vi "Dac_Voice_coil_Camera_trigger.vi"(0 "Voice coil function generation":T1={"File to read"=path "C:/Users/lpk27/Documents/pan-ASLMsynched/pan-ASLM/Calibration files/newcalibration_voice coil input_25msflyback.txt", "Image acquisition time (ms)"=1000.0, "Flyback time (ms)"=25.0}, 5 "error in":errorcluster, 9 "DAQ setup":enum16{"Test setup", "Microscope"}(ring)) -> ()   [LabVIEW 2020]
uses:
  typedefs/typedef_voice_coil_function_generation.ctl
  <vilib>/DAQmx/write.llb/DAQmx Write (Analog Wfm 1Chan NSamp).vi
  <vilib>/Utility/file.llb/Read Delimited Spreadsheet (DBL).vi
  <vilib>/DAQmx/create/channels.llb/DAQmx Create Channel (AO-Voltage-Basic).vi
  <vilib>/DAQmx/configure/timing.llb/DAQmx Timing (Sample Clock).vi
  <vilib>/DAQmx/miscellaneous.llb/DAQmx Fill In Error Info.vi
  <vilib>/DAQmx/create/channels.llb/DAQmx Create Channel (CO-Pulse Generation-Ticks).vi
  <vilib>/DAQmx/configure/timing.llb/DAQmx Timing (Implicit).vi
  <vilib>/DAQmx/create/channels.llb/DAQmx Create Channel (CO-Pulse Generation-Frequency).vi
  Global stop DAQ.vi
  <resource>/objmgr/daqmx.rc
panel:
  out "error out 4":errorcluster
  out "error out 3":errorcluster
  out "LabVIEW generated Sawtooth input (blue) and Camera trigger (red)":waveform(dbl)(graph)={"t0"=timestamp(0 s since 1904-01-01), "dt"=1.0, "Y"=array[3075 elements]}
  out "# Samples written per channel":u32=3075
  out "actual frequency":dbl=1000.0
  in  "stop":bool
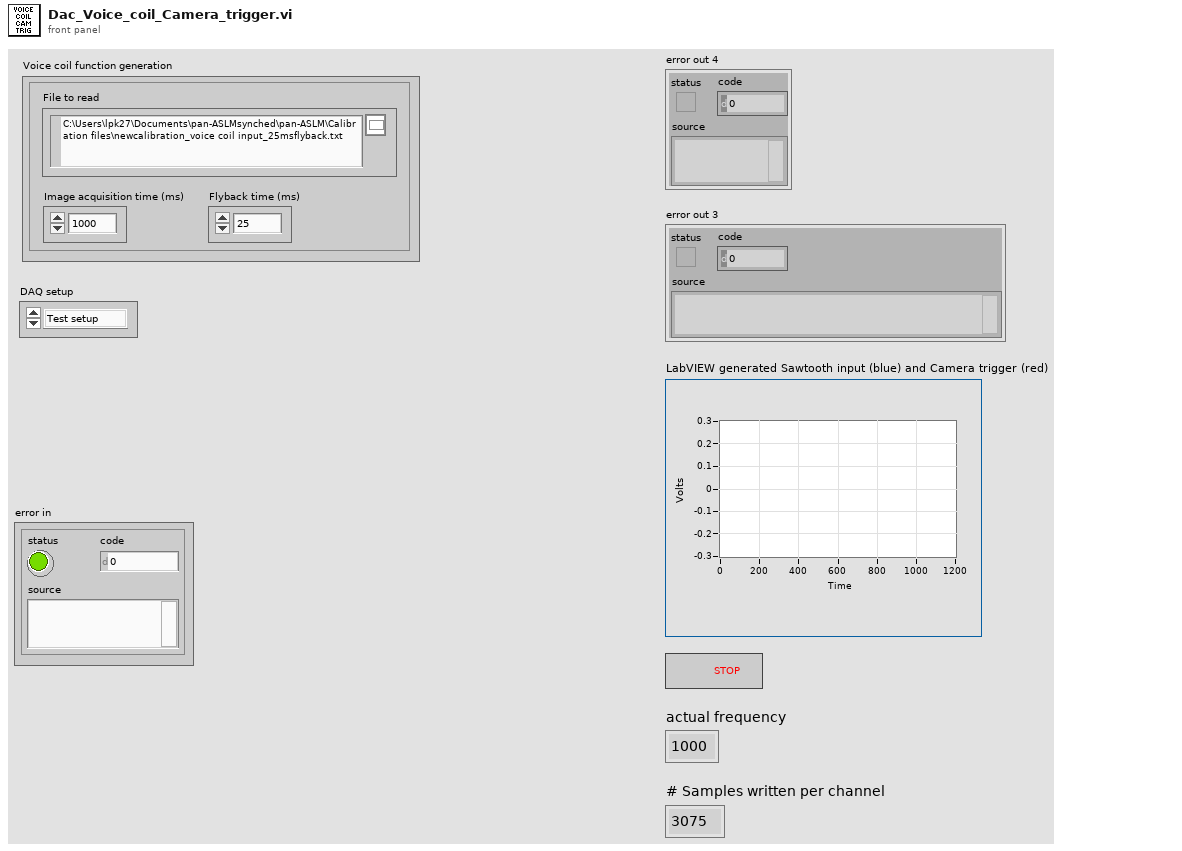
[diagram p1: front panel]
types:
  T1 = typedef "typedef_voice_coil_function_generation.ctl" = cluster{"File to read":path, "Image acquisition time (ms)":dbl, "Flyback time (ms)":dbl}
  T2 = typedef "DAQ_channel_typedef.ctl" = cluster{"CO.Pulse.Term":tag, "Voice coil analog output":tag, "counter":tag, "CO.Pulse.Term 2":tag, "AOTF lines":tag, "counter 2":tag, "CO.Pulse.Term 3":tag, "counter 3":tag}
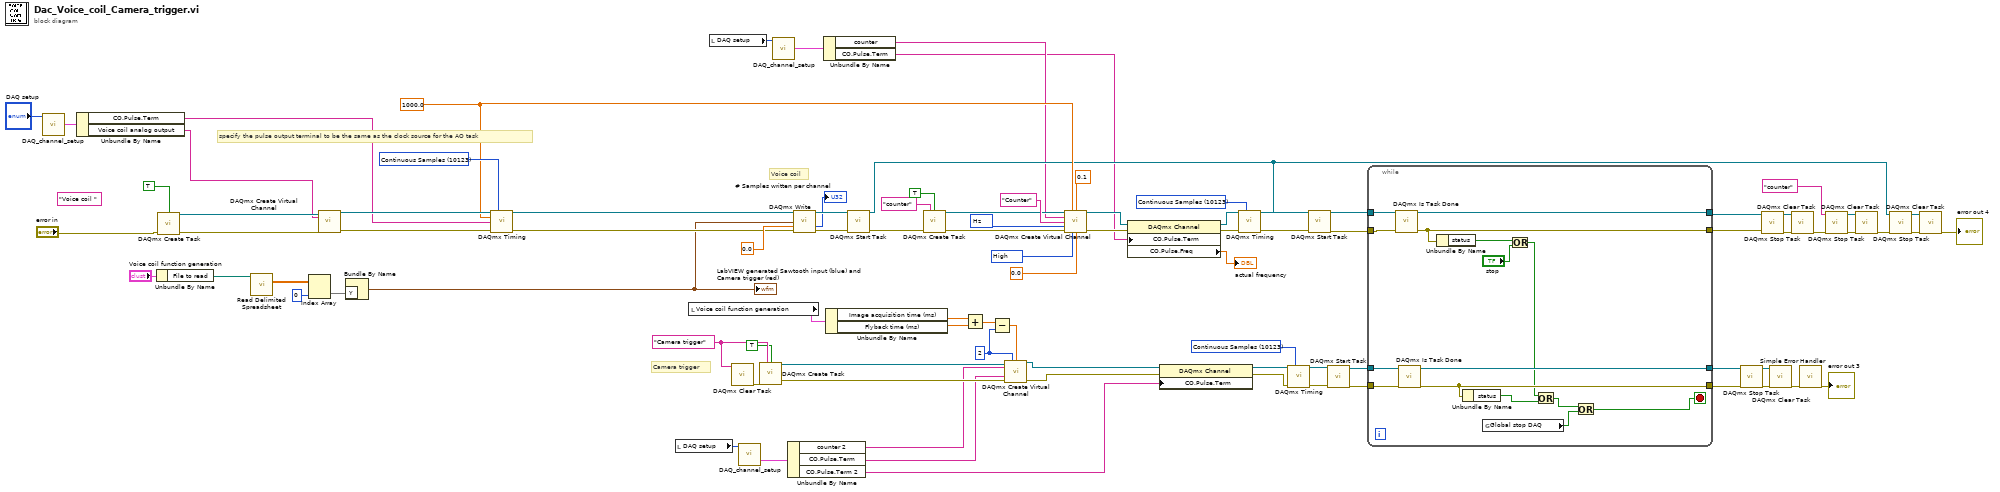
[diagram p0: block diagram]
diagram:
  w20 = "Camera trigger" ("new task name")
  (unwired) "Voice coil " ("new task name")
  w51 = u32 2 ("high ticks")
  w61 = 10123 items=["Finite Samples"=10178, "Continuous Samples"=10123, "Hardware Timed Single Point"=12522] ("sample mode")
  w73 = 10192 items=["High"=10192, "Low"=10214] ("idle state")
  w74 = 10373 items=["Hz"=10373] ("units")
  w67 = 10123 items=["Finite Samples"=10178, "Continuous Samples"=10123, "Hardware Timed Single Point"=12522] ("sample mode")
  w66 = 1000.0 ("rate")
  w89 = 10123 items=["Finite Samples"=10178, "Continuous Samples"=10123, "Hardware Timed Single Point"=12522] ("sample mode")
  # "Camera trigger"
  # "Voice coil"
  # "specify the pulse output terminal to be the same as the clock source for the AO task"
  n1 = call "DAQ_channel_setup.vi"("Text Ring"="DAQ setup") -> ("DAQ channels OUT"=w14:T2)  [unwired: 10 in]
  n2 = Unbundle By Name(w14) -> ("CO.Pulse.Term"=w4:tag, "Voice coil analog output"=w13:tag)
  n3 = Unbundle By Name("Voice coil function generation") -> ("File to read"=w44:path)
  n4 = call <vilib>:"DAQmx Create Task.vi"("auto cleanup"=TRUE, "error in"="error in") -> ("task out"=w49:refnum<k21>, "error out"=w48:errorcluster)  [unwired: 12 in]
  n5 = call-poly <vilib>:"Read Delimited Spreadsheet.vi"("file path (dialog if empty)"=w44) -> ("all rows"=w58:dbl[][])  [unwired: 9 in, 5 out]
  n6 = Index Array(array=w58, index (col)=0 ("disabled index (col)")) -> (element=w56:dbl[])  [unwired: 1 in]
  n7 = call-poly <vilib>:"DAQmx Create Virtual Channel.vi"("task in"=w49, "physical channels"=w13, "error in"=w48) -> ("task out"=w91:refnum<k21>, "error out"=w90:errorcluster)  [unwired: 11 in]
  n8 = Bundle By Name("Y"=w56) -> (w55:waveform(dbl))  [unwired: 1 in]
  "LabVIEW generated Sawtooth input (blue) and Camera trigger (red)" <- w55
  n9 = call-poly <vilib>:"DAQmx Timing.vi"("task/channels in"=w91, "sample mode"=w89, "rate"=w66, "source"=w4, "error in"=w90) -> ("task out"=w69:refnum<k21>, "error out"=w68:errorcluster)  [unwired: 9 in]
  n10 = local read "DAQ setup"() -> (w11:enum16{"Test setup", "Microscope"})
  n11 = local read "Voice coil function generation"() -> (w43:T1)
  n12 = local read "DAQ setup"() -> (w7:enum16{"Test setup", "Microscope"})
  n13 = call <vilib>:"DAQmx Clear Task.vi"("task in"=w20) -> ("error out"=w21:errorcluster)  [unwired: 14 in]
  n14 = call "DAQ_channel_setup.vi"("Text Ring"=w11) -> ("DAQ channels OUT"=w12:T2)  [unwired: 10 in]
  n15 = call <vilib>:"DAQmx Create Task.vi"("new task name"=w20, "auto cleanup"=TRUE, "error in"=w21) -> ("task out"=w46:refnum<k21>, "error out"=w47:errorcluster)  [unwired: 11 in]
  n16 = call "DAQ_channel_setup.vi"("Text Ring"=w7) -> ("DAQ channels OUT"=w6:T2)  [unwired: 10 in]
  n17 = Unbundle By Name(w12) -> ("counter 2"=w10:tag, "CO.Pulse.Term"=w9:tag, "CO.Pulse.Term 2"=w8:tag)
  n18 = call-poly <vilib>:"DAQmx Write.vi"("task/channels in"=w69, "data"=w55, "timeout"=0.0, "error in"=w68) -> ("task out"=w78:refnum<k21>, "number of samples written per channel"=→"# Samples written per channel":u32, "error out"=w77:errorcluster)  [unwired: 9 in]
  n19 = Unbundle By Name(w6) -> ("counter"=w5:tag, "CO.Pulse.Term"=w3:tag)
  n20 = Unbundle By Name(w43) -> ("Image acquisition time (ms)"=w42:dbl, "Flyback time (ms)"=w41:dbl)
  n21 = call <vilib>:"DAQmx Start Task.vi"("task/channels in"=w78, "error in"=w77) -> ("task out"=w33:refnum<k21>, "error out"=w72:errorcluster)  [unwired: 12 in]
  n22 = call <vilib>:"DAQmx Create Task.vi"("new task name"="counter", "auto cleanup"=TRUE, "error in"=w72) -> ("task out"=w28:refnum<k21>, "error out"=w85:errorcluster)  [unwired: 11 in]
  n23 = Add(x=w42, y=w41) -> (x+y=w52:dbl)
  n24 = Subtract(x=w52, y=w51) -> (x-y=w50:dbl)
  n25 = call-poly <vilib>:"DAQmx Create Virtual Channel.vi"("task in"=w46, "high ticks"=w51, "low ticks"=w50, "counter"=w10, "source of ticks"=w9, "error in"=w47) -> ("task out"=w65:refnum<k21>, "error out"=w54:errorcluster)  [unwired: 8 in]
  n26 = call-poly <vilib>:"DAQmx Create Virtual Channel.vi"("task in"=w28, "frequency"=w66, "duty cycle"=0.1, "counter"=w5, "name to assign"="Counter", "units"=w74, "error in"=w85, "idle state"=w73, "initial delay"=0.0) -> ("task out"=w84:refnum<k21>, "error out"=w83:errorcluster)  [unwired: 5 in]
  n27 = property class="DAQmx Channel"(reference=w84, error in=w83, "CO.Pulse.Term"=w3) -> (reference out=w80:refnum<k21>, error out=w81:errorcluster, "CO.Pulse.Freq"=→"actual frequency":dbl)
  n28 = property class="DAQmx Channel"(reference=w65, error in=w54, "CO.Pulse.Term"=w8) -> (reference out=w53:refnum<k21>, error out=w62:errorcluster)
  n29 = call-poly <vilib>:"DAQmx Timing.vi"("task/channels in"=w80, "sample mode"=w67, "error in"=w81) -> ("task out"=w88:refnum<k21>, "error out"=w87:errorcluster)  [unwired: 11 in]
  n30 = call-poly <vilib>:"DAQmx Timing.vi"("task/channels in"=w53, "sample mode"=w61, "error in"=w62) -> ("task out"=w60:refnum<k21>, "error out"=w59:errorcluster)  [unwired: 11 in]
  n31 = call <vilib>:"DAQmx Start Task.vi"("task/channels in"=w88, "error in"=w87) -> ("error out"=w79:errorcluster)  [unwired: 12 in, 1 out]
  n32 = call <vilib>:"DAQmx Start Task.vi"("task/channels in"=w60, "error in"=w59) -> ("task out"=w64:refnum<k21>, "error out"=w63:errorcluster)  [unwired: 12 in]
  n33 = while {
    tunnel: w79 -> [w106]
    tunnel: w33 -> [w105]
    tunnel: w64 -> [w104]
    tunnel: w63 -> [w103]
    tunnel: [w100] -> w35
    tunnel: [w99] -> w34
    tunnel: [w98] -> w23
    tunnel: [w97] -> w22
    stop <- w92 stop-if-true
    n34 = call <vilib>:"DAQmx Is Task Done.vi"("task/channels in"=w105, "error in"=w106) -> ("task out"=w100:refnum<k21>, "error out"=w99:errorcluster)  [unwired: 11 in, 1 out]
    n35 = call <vilib>:"DAQmx Is Task Done.vi"("task/channels in"=w104, "error in"=w103) -> ("task out"=w98:refnum<k21>, "error out"=w97:errorcluster)  [unwired: 11 in, 1 out]
    n36 = Unbundle By Name(w99) -> ("status"=w102:bool)
    n37 = Unbundle By Name(w97) -> ("status"=w96:bool)
    n38 = global read "Global stop DAQ.vi" "Global stop DAQ"() -> (w93:bool)
    n39 = Or(x=w102, y="stop") -> (x .or. y?=w95:bool)
    n40 = Or(x=w95, y=w96) -> (x .or. y?=w94:bool)
    n41 = Or(x=w94, y=w93) -> (x .or. y?=w92:bool)
  }
  n42 = call <vilib>:"DAQmx Stop Task.vi"("task/channels in"=w23, "error in"=w22) -> ("task out"=w26:refnum<k21>, "error out"=w27:errorcluster)  [unwired: 12 in]
  n43 = call <vilib>:"DAQmx Stop Task.vi"("task/channels in"=w35, "error in"=w34) -> ("task out"=w38:refnum<k21>, "error out"=w37:errorcluster)  [unwired: 12 in]
  n44 = call <vilib>:"DAQmx Clear Task.vi"("task in"=w26, "error in"=w27) -> ("error out"=w25:errorcluster)  [unwired: 13 in]
  n45 = call <vilib>:"DAQmx Clear Task.vi"("task in"=w38, "error in"=w37) -> ("error out"=w29:errorcluster)  [unwired: 13 in]
  n46 = call <vilib>:"Simple Error Handler.vi"("error in (no error)"=w25) -> ("error out"=→"error out 3":errorcluster)  [unwired: 4 in, 4 out]
  n47 = call <vilib>:"DAQmx Stop Task.vi"("task/channels in"="counter" ("new task name"), "error in"=w29) -> ("task out"=w32:refnum<k21>, "error out"=w31:errorcluster)  [unwired: 12 in]
  n48 = call <vilib>:"DAQmx Clear Task.vi"("task in"=w32, "error in"=w31) -> ("error out"=w30:errorcluster)  [unwired: 13 in]
  n49 = call <vilib>:"DAQmx Stop Task.vi"("task/channels in"=w33, "error in"=w30) -> ("task out"=w39:refnum<k21>, "error out"=w40:errorcluster)  [unwired: 12 in]
  n50 = call <vilib>:"DAQmx Clear Task.vi"("task in"=w39, "error in"=w40) -> ("error out"=→"error out 4":errorcluster)  [unwired: 13 in]
